vi "Reorder Views.vi"(8 "error in (no error)":errorcluster, 11 "SubPanel Grid View in":refnum<class "SubPanel Grid View.lvclass">) -> (0 "error out":errorcluster, 3 "SubPanel Grid View out":refnum<class "SubPanel Grid View.lvclass">)   [LabVIEW 2012, in "Win8uiDemo.lvlib" / "SubPanel Grid View.lvclass"]
uses:
  SubPanel Grid View.lvclass
  SubPanel Grid View.lvclass/SubPanel Grid View.ctl
  <vilib>/ActorFramework/Message Enqueuer/Message Enqueuer.lvclass/Message Enqueuer.ctl
  SubPanel 3x3 View/Read SubPanel Array.vi
  Read ViewableActor Enqueuers.vi
  Write NextIndex.vi
  <vilib>/ActorFramework/Message Enqueuer/Enqueue.vi
  <vilib>/ActorFramework/Message Priority Queue/Priority Enqueue.vi
  <vilib>/ActorFramework/Message Enqueuer/Message Enqueuer.lvclass
  Win8uiFramework/Remove From SubPanel Msg.lvclass
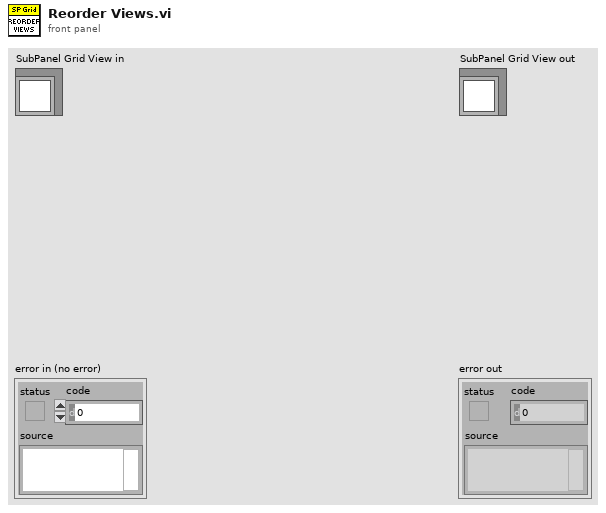
[diagram p1: front panel]
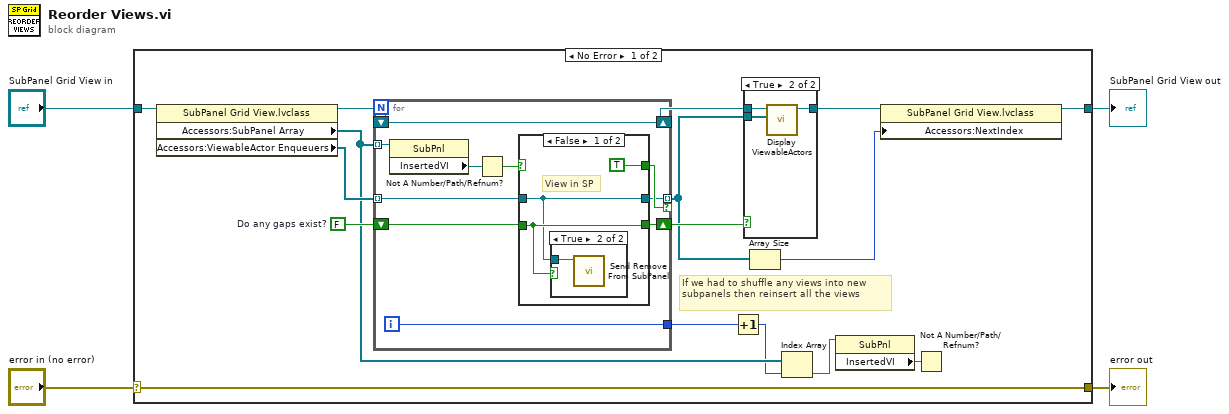
[diagram p0: block diagram]
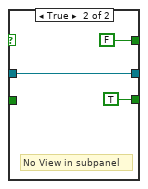
[diagram p4: hidden frame]
diagram:
  n1 = case shown="No Error" "error in (no error)" {
    selector: "error in (no error)" -> [w19 w43]
    tunnel: [w19 w43] -> w3
    tunnel: [w12 w42] -> w1
    tunnel: "SubPanel Grid View in" -> [w20 w42]
    frame No Error {
      w16 = FALSE  # Do any gaps exist?
      # "If we had to shuffle any views into new subpanels then reinsert all the views"
      n2 = property class="SubPanel Grid View.lvclass"(reference=w20) -> (reference out=w18:refnum<class "SubPanel Grid View.lvclass">, "Accessors:SubPanel Array"=w8:refnum<vi>[], "Accessors:ViewableActor Enqueuers"=w17:refnum<class "Message Enqueuer.lvclass">[])  [unwired: 1 in, 1 out]
      n3 = for {
        tunnel: w8 -> [w33] mode=indexing
        shift-right: [w34] -> w15
        shift-left: w18 -> [w34]
        shift-right: [w29] -> w13
        shift-left: w16 -> [w28]
        tunnel: w17 -> [w30] mode=indexing
        tunnel: [w26] -> w11 mode=indexing if=w27
        tunnel: [w25] -> w9
        i -> [w25]
        n4 = property class="SubPnl"(reference=w33) -> ("InsertedVI"=w32:refnum<vi>)  [unwired: 1 in, 2 out]
        n5 = Not A Number/Path/Refnum?(number/path/refnum=w32) -> (NaN/Path/Refnum?=w31:bool)
        n6 = case shown="False" w31 {
          tunnel: w30 -> [w35 w40]
          tunnel: [w36 TRUE] -> w29
          tunnel: w28 -> [w36 _]
          tunnel: [TRUE FALSE] -> w27
          tunnel: [w35 w40] -> w26
          frame False {
            # "View in SP"
            n7 = case shown="True" w36 {
              tunnel: w35 -> [_ w38]
              frame False {
              }
              frame True {
                n8 = call "Send Remove From SubPanel.vi"("Message Enqueuer"=w38) -> ()  [unwired: 9 in, 2 out]
              }
            }
          }
          frame True {
            # "No View in subpanel"
          }
        }
      }
      n9 = Increment(x=w9) -> (x+1=w7:i32)
      n10 = case shown="True" w13 {
        tunnel: w15 -> [w21 w24]
        tunnel: [w21 w23] -> w14
        tunnel: w11 -> [_ w22]
        frame False {
        }
        frame True {
          n11 = call-dynamic "Display ViewableActors.vi"("ViewableActor Enqueuers"=w22, "SubPanel Grid View in"=w24) -> ("SubPanel Grid View out"=w23:refnum<class "SubPanel Grid View.lvclass">)  [unwired: 8 in, 1 out]
        }
      }
      n12 = Array Size(array=w11) -> (size(s)=w10:i32)
      n13 = Index Array(array=w8, index=w7) -> (element=w6:refnum<vi>)
      n14 = property class="SubPnl"(reference=w6) -> ("InsertedVI"=w5:refnum<vi>)  [unwired: 1 in, 2 out]
      n15 = property class="SubPanel Grid View.lvclass"(reference=w14, "Accessors:NextIndex"=w10) -> (reference out=w12:refnum<class "SubPanel Grid View.lvclass">)  [unwired: 1 in, 1 out]
      n16 = Not A Number/Path/Refnum?(number/path/refnum=w5) -> ()  [unwired: 1 out]
    }
    frame Error {
    }
  }
  "error out" <- w3
  "SubPanel Grid View out" <- w1
